vi "TestACPad.vi"() -> ()   [LabVIEW 2018]
uses:
  <vilib>/Utility/file.llb/Read Delimited Spreadsheet (DBL).vi
panel:
  in  "AC Pad #":i32
  in  "Move to Position":bool
  in  "stop":bool
  # "Moves to the index specified by \"AC Pad #\" after pressing \"Move to Position\". Pressing \"Stop\" \nends the program but will not halt movement. Movement is observed with the Vision module."
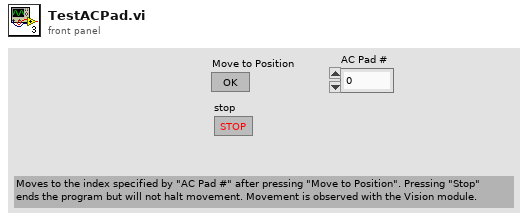
[diagram p1: front panel]
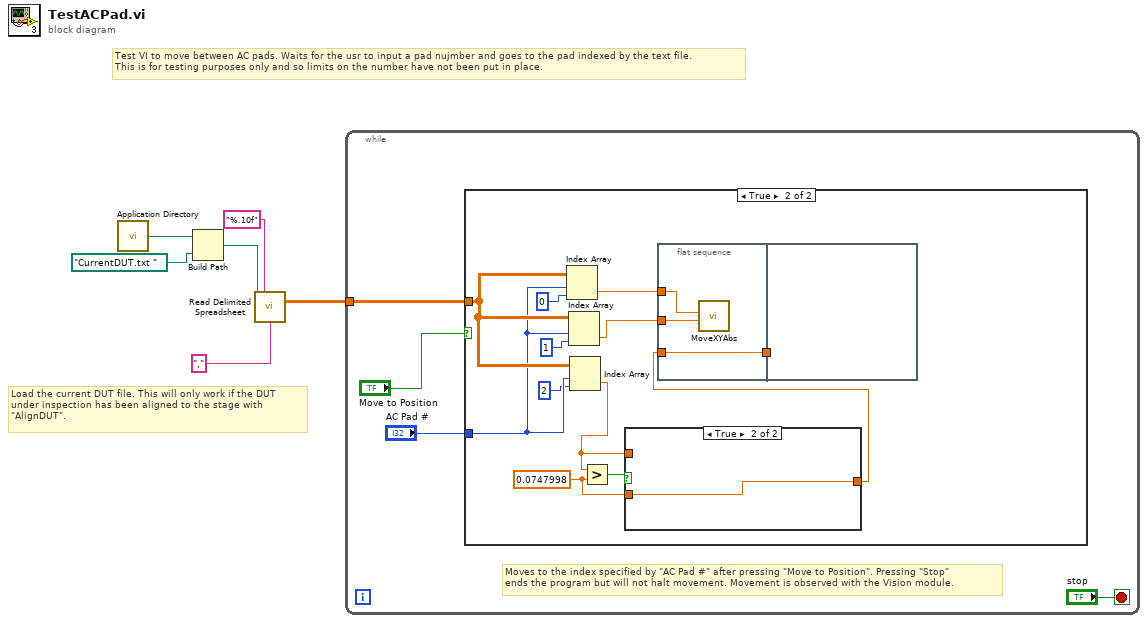
[diagram p0: block diagram]
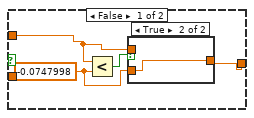
[diagram p3: hidden frame]
diagram:
  # "Load the current DUT file. This will only work if the DUT \nunder inspection has been aligned to the stage with \n\"AlignDUT\"."
  # "Test VI to move between AC pads. Waits for the usr to input a pad nujmber and goes to the pad indexed by the text file. \nThis is for testing purposes only and so limits on the number have not been put in place."
  n1 = call <vilib>:"Application Directory.vi"() -> ("Application Directory"=w3:path)
  n2 = Build Path(base path=w3, name or relative path=path "CurrentDUT.txt " ("file path (dialog if empty)")) -> (appended path=w4:path)
  n3 = call-poly <vilib>:"Read Delimited Spreadsheet.vi"("file path (dialog if empty)"=w4, "format (%.3f)"="%.10f", "delimiter (\\t)"="," ("delimiter (\\t)")) -> ("all rows"=w1:dbl[][])  [unwired: 7 in, 5 out]
  n4 = while {
    tunnel: w1 -> [w8]
    stop <- "stop" stop-if-true
    # "Moves to the index specified by \"AC Pad #\" after pressing \"Move to Position\". Pressing \"Stop\" \nends the program but will not halt movement. Movement is observed with the Vision module."
    n5 = case shown="True" "Move to Position" {
      tunnel: w8 -> [_ w22]
      tunnel: "AC Pad #" -> [_ w21]
      frame False {
      }
      frame True {
        w16 = 0.0747998 ("y")
        n6 = Index Array(array=w22, index (row)=w21, index (col)=0 ("disabled index (col)")) -> (element=w14:dbl)
        n7 = Index Array(array=w22, index (row)=w21, index (col)=1 ("disabled index (col)")) -> (element=w13:dbl)
        n8 = Index Array(array=w22, index (row)=w21, index (col)=2 ("disabled index (col)")) -> (element=w15:dbl)
        n9 = Greater?(x=w15, y=w16) -> (0:w17:bool)
        n10 = case shown="True" w17 {
          tunnel: [w29 w32] -> w11
          tunnel: w16 -> [_ w32]
          tunnel: w15 -> [w28 _]
          frame False {
            w26 = -0.0747998 ("y")
            n11 = Less?(x=w28, y=w26) -> (x < y?=w27:bool)
            n12 = case shown="True" w27 {
              tunnel: w28 -> [w30 _]
              tunnel: [w30 w31] -> w29
              tunnel: w26 -> [_ w31]
              frame False {
              }
              frame True {
              }
            }
          }
          frame True {
          }
        }
        n13 = flat-sequence {
          tunnel: w14 -> [w25]
          tunnel: w13 -> [w24]
          tunnel: w11 -> [w23]
          tunnel: [w23] -> w12
          tunnel: w12 -> [_]
          frame #0 {
            n14 = call "MoveXYAbs.vi"("Y"=w24, "X"=w25) -> ()  [unwired: 9 in, 1 out]
          }
          frame #1 {
          }
        }
      }
    }
  }
